vi "Análise de Sinais - Turma 07 - Grupo 05 - MatheusRibeiro_11261103.vi"(8 "Error In":errorcluster) -> (0 "Error Out":errorcluster)   [LabVIEW 2014]
uses:
  <vilib>/Waveform/WDTOps.llb/WDT Waveform Duration DBL.vi
  <vilib>/Waveform/WDTOps.llb/WDT Number of Waveform Samples DBL.vi
  <vilib>/measure/mascope.llb/Amplitude and Levels 1 chan.vi
  <vilib>/express/express analysis/Spectral/Block/exnSpectralBlock spectral measurements peak poly.vi
  <vilib>/express/express analysis/Spectral/Block/exnSpectralBlock spectral measurements peak WFM.vi
  <vilib>/express/express analysis/Spectral/XNode/ExpressSpectralMeasurementsBlockNode.xnode
  Aquisicao de Dados.lvlib
  <vilib>/measure/NI_MAPro.lvlib
panel:
  out "Canal 0":waveform(dbl)(graph)
  out "Resolução de Frequência":dbl
  out "Frequência Associada":dbl
  out "Maior Amplitude":dbl
  out "Período Amostral (s)":dbl
  out "Frequência Amostral (Hz)":dbl
  out "Número Amostral":dbl
  out "Amplitude do Sinal (%)":dbl
  out "Espectro do Canal 0":cluster{"f0":dbl, "df":dbl, "magnitude":dbl[]}(graph)
  out "Espectro do Canal 1":cluster{"f0":dbl, "df":dbl, "magnitude":dbl[]}(graph)
  out "Resolução de Frequência":dbl
  out "Frequência Associada":dbl
  out "Maior Amplitude":dbl
  out "Período Amostral (s)":dbl
  out "Frequência Amostral (Hz)":dbl
  out "Número Amostral":dbl
  out "Amplitude do Sinal (%)":dbl
  out "Canal 1":waveform(dbl)(graph)
  # "Dados do Sinal do Canal 0"
  # "Dados do Sinal do Canal 1"
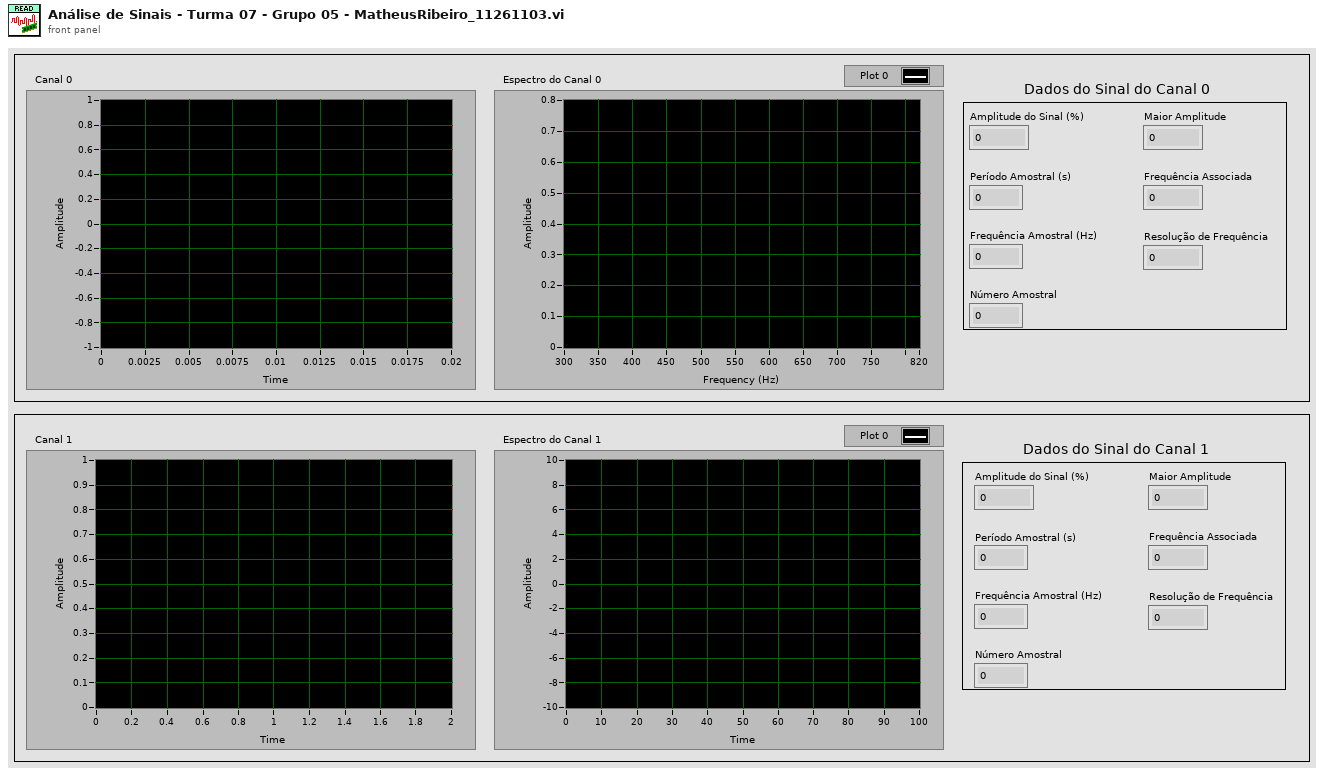
[diagram p1: front panel]
types:
  T1 = enum32{".WAV File", "LTSpice Simulation", "Microphone", "MultiSim Simulation", "Serial Port"}
  T2 = typedef "Aquisicao de Dados.lvlib/_ACC_DATA_ Config DAta State.ctl" = cluster{"_RAW_ Traces":cluster{"Trace Name":string, "Trace Type":string, "Trace Raw Data":dbl[], "Trace Waveform":waveform(dbl)}[], "_WAV_ Traces":waveform(dbl)[], "_MIC_ Config":cluster{"task ID":T3, "Data Chunk Size":i32, "Num Channels":i32, "Resolution":i32, "Sampling Frequency":dbl, "device ID":u32, "Num Chunks":i32}, "_LVM_ Traces":cluster{"Trace Name":string, "Trace Type":string, "Trace Raw Data":dbl[], "Trace Waveform":waveform(dbl)}[]}
  T3 = typedef "Sound Input Task ID.ctl" = u32
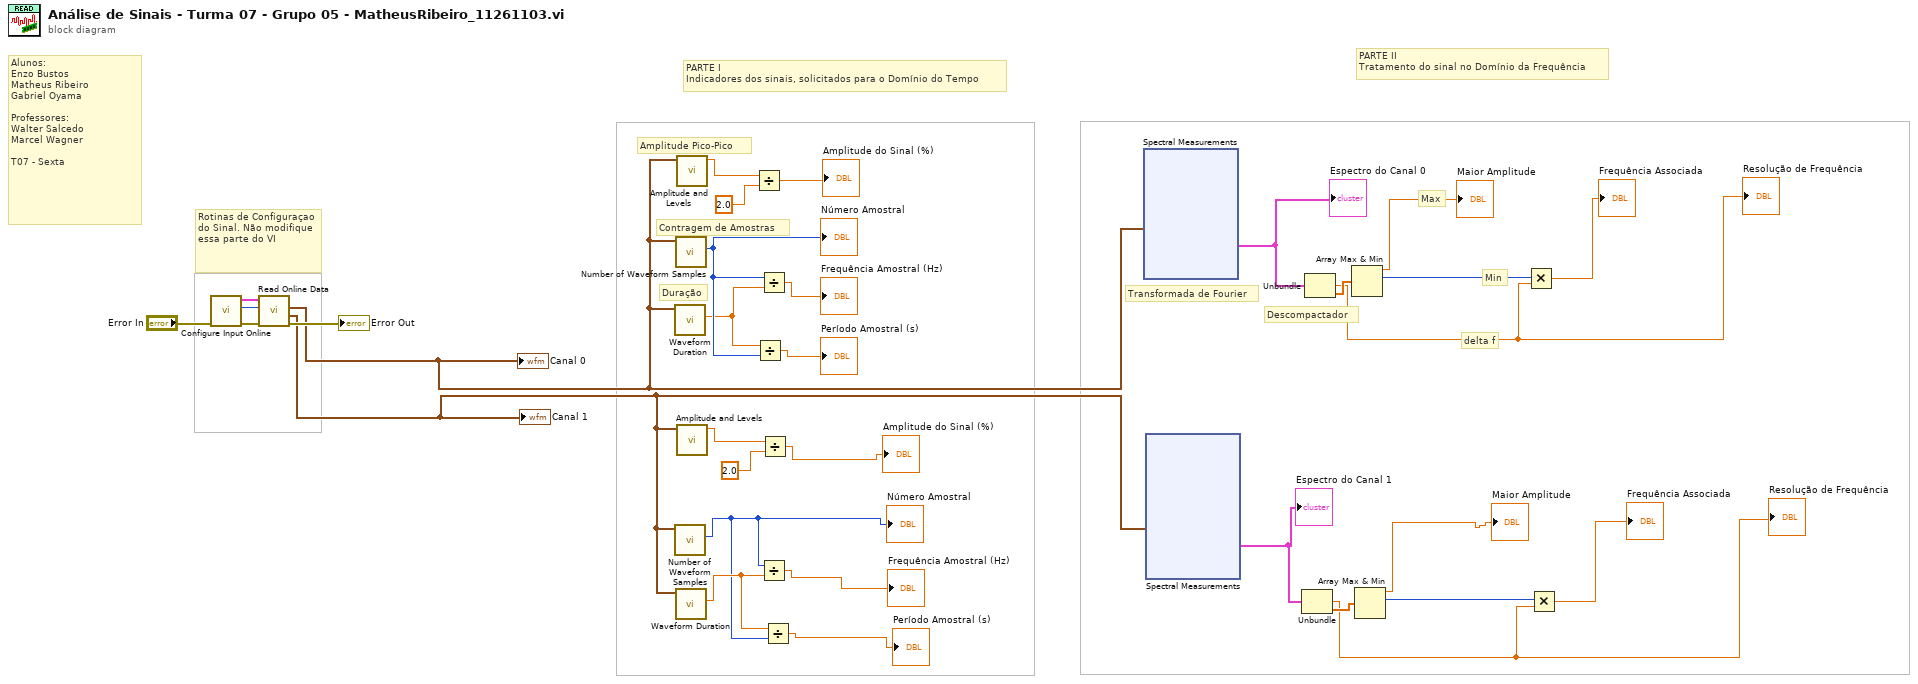
[diagram p0: block diagram]
diagram:
  # "Alunos:\nEnzo Bustos\nMatheus Ribeiro\nGabriel Oyama\n\nProfessores:\nWalter Salcedo\nMarcel Wagner\n\nT07 - Sexta"
  # "delta f"
  # "Min"
  # "Max"
  # "Descompactador"
  # "Transformada de Fourier"
  # "Duração"
  # "Contragem de Amostras"
  # "Amplitude Pico-Pico"
  # "PARTE II\nTratamento do sinal no Domínio da Frequência"
  # "PARTE I\nIndicadores dos sinais, solicitados para o Domínio do Tempo"
  # "Rotinas de Configuraçao do Sinal. Não modifique essa parte do VI"
  n1 = call "Configure Input Online.vi"("Error In"="Error In") -> ("Error Out"=w33:errorcluster, "Metodo de Entrada"=w31:T1, "Config Out"=w29:T2)  [unwired: 8 in]
  n2 = call "Read Online Data.vi"("Error In"=w33, "Metodo de Entrada"=w31, "Config Out"=w29) -> ("Error Out"=→"Error Out":errorcluster, "Channel 1"=w2:waveform(dbl), "Channel 0"=w1:waveform(dbl))  [unwired: 6 in]
  "Canal 1" <- w2
  "Canal 0" <- w1
  n3 = call-poly <vilib>:"Waveform Duration.vi"("waveform in"=w1) -> ("duration"=w22:dbl)  [unwired: 8 in, 2 out]
  n4 = call-poly <vilib>:"Number of Waveform Samples.vi"("waveform in"=w2) -> ("number of samples"=w8:i32)  [unwired: 8 in, 2 out]
  "Número Amostral" <- w8
  n5 = call-poly <vilib>:"Number of Waveform Samples.vi"("waveform in"=w1) -> ("number of samples"=w23:i32)  [unwired: 8 in, 2 out]
  "Número Amostral" <- w23
  n6 = call-poly <vilib>:"Waveform Duration.vi"("waveform in"=w2) -> ("duration"=w19:dbl)  [unwired: 8 in, 2 out]
  n7 = call-poly <vilib>:"Amplitude and Levels.vi"("signal in"=w1) -> ("amplitude"=w27:dbl)  [unwired: 7 in, 3 out]
  n8 = call-poly <vilib>:"Amplitude and Levels.vi"("signal in"=w2) -> ("amplitude"=w25:dbl)  [unwired: 7 in, 3 out]
  n9 = Divide(x=w27, y=2.0) -> (x/y=→"Amplitude do Sinal (%)":dbl)
  n10 = Divide(x=w22, y=w23) -> (x/y=→"Período Amostral (s)":dbl)
  n11 = Divide(x=w23, y=w22) -> (x/y=→"Frequência Amostral (Hz)":dbl)
  n12 = Divide(x=w8, y=w19) -> (x/y=→"Frequência Amostral (Hz)":dbl)
  n13 = Divide(x=w25, y=2.0) -> (x/y=→"Amplitude do Sinal (%)":dbl)
  n14 = Divide(x=w19, y=w8) -> (x/y=→"Período Amostral (s)":dbl)
  n15 = xnode "Spectral Measurements"("Signals"=w1) -> ("FFT - (Peak)"=w10:cluster{"f0":dbl, "df":dbl, "magnitude":dbl[]})  [unwired: 1 in, 2 out]
  "Espectro do Canal 0" <- w10
  n16 = xnode "Spectral Measurements"("Signals"=w2) -> ("FFT - (Peak)"=w14:cluster{"f0":dbl, "df":dbl, "magnitude":dbl[]})  [unwired: 1 in, 2 out]
  "Espectro do Canal 1" <- w14
  n17 = Unbundle(w14) -> ("df"=w5:dbl, "magnitude"=w13:dbl[])  [unwired: 1 out]
  "Resolução de Frequência" <- w5
  n18 = Unbundle(w10) -> ("df"=w11:dbl, "magnitude"=w12:dbl[])  [unwired: 1 out]
  "Resolução de Frequência" <- w11
  n19 = Array Max & Min(array=w12) -> (max value=→"Maior Amplitude":dbl, max index (indices)=w17:i32)  [unwired: 2 out]
  n20 = Array Max & Min(array=w13) -> (max value=→"Maior Amplitude":dbl, max index (indices)=w15:i32)  [unwired: 2 out]
  n21 = Multiply(x=w17, y=w11) -> (x*y=→"Frequência Associada":dbl)
  n22 = Multiply(x=w15, y=w5) -> (x*y=→"Frequência Associada":dbl)
